vi "WSVCAP SHL Host TL Initialize.vi"(11 "error in":errorcluster, 14 "FPGA":T1) -> (4 "System":T2={"Settings"={"I2C Slave Address"=144, "I2C Clock Rate (Hz)"=20.0, "SRL Clock Rate (Hz)"=50000.0, "Simulate FPGA"=TRUE, "C1 Cap DAC Default"=165, "C2 Cap DAC Default"=165, "C3 Cap DAC Default"=134, "C4 Cap DAC Default"=150, "DAC Out Vref (V)"=0.0}, "FPGA Resource"="", "Online"=FALSE, "I2C Wait Ticks"=0, "SRL Wait Ticks"=0, "FPGA VI Reference (FPGA Mode)"=refnum, "FPGA VI Reference (Sim Mode)"=refnum} {"Settings"."DAC Out Vref (V)" format="%.3f V"; "Settings"."C4 Cap DAC Default" format="0x%02x"; "Settings"."C3 Cap DAC Default" format="0x%02x"; "Settings"."C2 Cap DAC Default" format="0x%02x"; "Settings"."C1 Cap DAC Default" format="0x%02x"; "Settings"."SRL Clock Rate (Hz)" format="%.0f Hz"; "Settings"."I2C Clock Rate (Hz)" format="%.0f Hz"; "Settings"."I2C Slave Address" format="0x%02x"}, 15 "error out":errorcluster)   [LabVIEW 2017]
uses:
  Type Defs/WSVCAP SHL Core System Cluster.ctl
  Type Defs/WSVCAP SHL I2C Settings Cluster.ctl
  Type Defs/WSVCAP SHL FPGA Ref.ctl
  Type Defs/WSVCAP SHL FPGA Enum.ctl
  Type Defs/WSVCAP SHL Function Enum.ctl
  Type Defs/WSVCAP SHL Gatekeeper Operation Enum.ctl
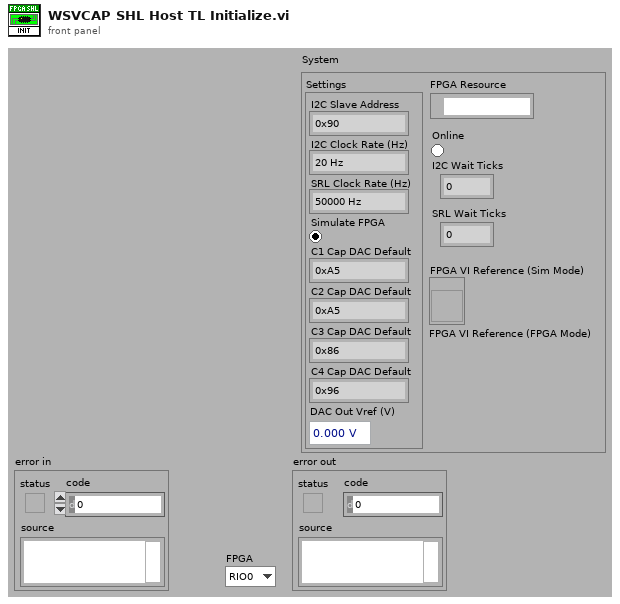
[diagram p1: front panel]
types:
  T1 = typedef "WSVCAP SHL FPGA Enum.ctl" = enum16{"RIO0", "RIO1"}
  T2 = typedef "WSVCAP SHL Core System Cluster.ctl" = cluster{"Settings":T3, "FPGA Resource":tag, "Online":bool, "I2C Wait Ticks":u32, "SRL Wait Ticks":u32, "FPGA VI Reference (FPGA Mode)":T4, "FPGA VI Reference (Sim Mode)":refnum<vi>}
  T3 = typedef "WSVCAP SHL I2C Settings Cluster.ctl" = cluster{"I2C Slave Address":u8, "I2C Clock Rate (Hz)":dbl, "SRL Clock Rate (Hz)":dbl, "Simulate FPGA":bool, "C1 Cap DAC Default":u8, "C2 Cap DAC Default":u8, "C3 Cap DAC Default":u8, "C4 Cap DAC Default":u8, "DAC Out Vref (V)":dbl}
  T4 = typedef "WSVCAP SHL FPGA Ref.ctl" = refnum<k20>
  T5 = typedef "WSVCAP SHL Gatekeeper Operation Enum.ctl" = enum16{"Initialize", "Lock", "Unlock", "Close"}
  T6 = typedef "WSVCAP SHL Function Enum.ctl" = enum16{"Initialize", "Configure I2C", "Configure SRL", "Write I2C", "Read I2C", "Write SRL", "Start SRL Cycle", "Stop SRL Cycle", "Get Status", "Close"}
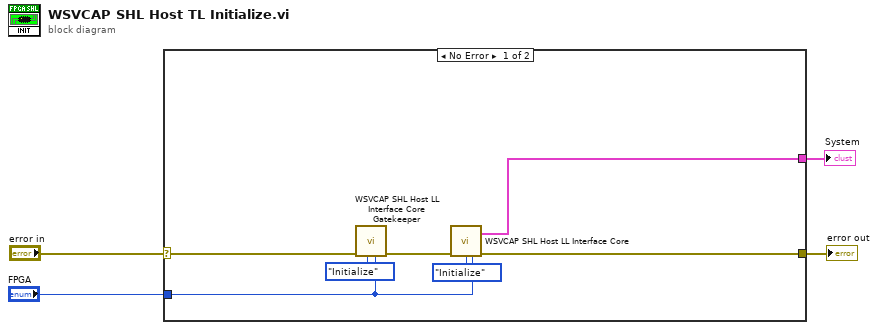
[diagram p0: block diagram]
diagram:
  n1 = case shown="No Error" "error in" {
    selector: "error in" -> [w7 w12]
    tunnel: [w11 w12] -> w3
    tunnel: [w9 _] -> w2
    tunnel: "FPGA" -> [w5 _]
    frame No Error {
      n2 = call "WSVCAP SHL Host LL Interface Core Gatekeeper.vi"("FPGA"=w5, "Operation"=WSVCAP_SHL_Gatekeeper_Operation_Enum."Initialize", "error in (no error)"=w7) -> ("error out"=w6:errorcluster)  [unwired: 8 in]
      n3 = call "WSVCAP SHL Host LL Interface Core.vi"("error in"=w6, "Function"=WSVCAP_SHL_Function_Enum."Initialize", "FPGA"=w5) -> ("System"=w9:T2, "error out"=w11:errorcluster)  [unwired: 10 in, 1 out]
    }
    frame Error {
    }
  }
  "error out" <- w3
  "System" <- w2
